vi "Get Raw Data.vi"(8 "error in (no error)":errorcluster, 11 "Red Pitaya Digitizer in":refnum<class "Red Pitaya Digitizer.lvclass">) -> (0 "error out":errorcluster, 1 "appended array":i16[][](array[numeric]), 3 "Red Pitaya Digitizer out":refnum<class "Red Pitaya Digitizer.lvclass">)   [LabVIEW 2021, in "Red Pitaya Digitizer.lvclass"]
uses:
  Red Pitaya Digitizer.lvclass
  C:/GitHub/NHMFL_Core/Libraries/Instruments/Pulse Driver/Lockin Digitizer Driver/Lockin Digitizer Driver.lvclass
  C:/GitHub/NHMFL_Core/Libraries/Instruments/Pulse Driver/Pulse Driver.lvclass
  Red Pitaya Digitizer.lvclass/Red Pitaya Digitizer.ctl
  Instruments/Pulse Driver/Pulse Driver.lvclass/Pulse Driver.ctl
  Read RP Instrument.vi
  Instruments/Pulse Driver/Read Pretrigger samples.vi
  Instruments/Pulse Driver/Read Samples per channel.vi
  Write RP Instrument.vi
  RP Core/RP Instrument/RP Instrument.lvclass
  Controls/Record Channels.ctl
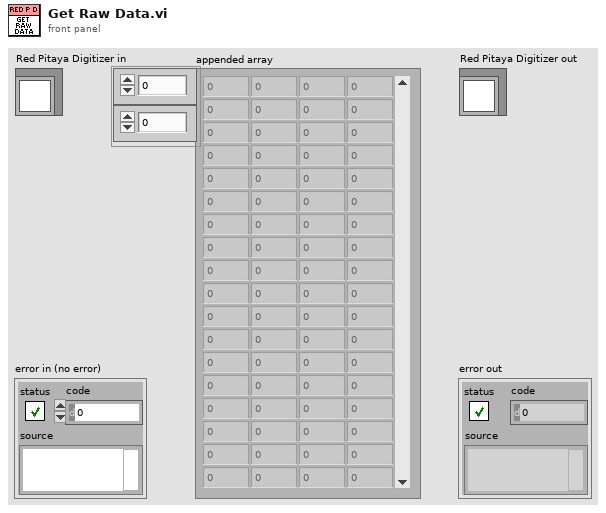
[diagram p1: front panel]
types:
  T1 = typedef "Record Channels.ctl" = enum16{"NONE", "FIRST", "SECOND", "BOTH"}
  T2 = enum16{"big-endian, network order", "native, host order", "little-endian"}
  T3 = typedef "Pusle Driver Configuration.ctl" = cluster{"Post-trigger delay":dbl, "Post-trigger duration":dbl, "Rate":dbl, "Ranges":dbl[], "Re-name channels":string[], "Active channels":string, "External clock":bool}
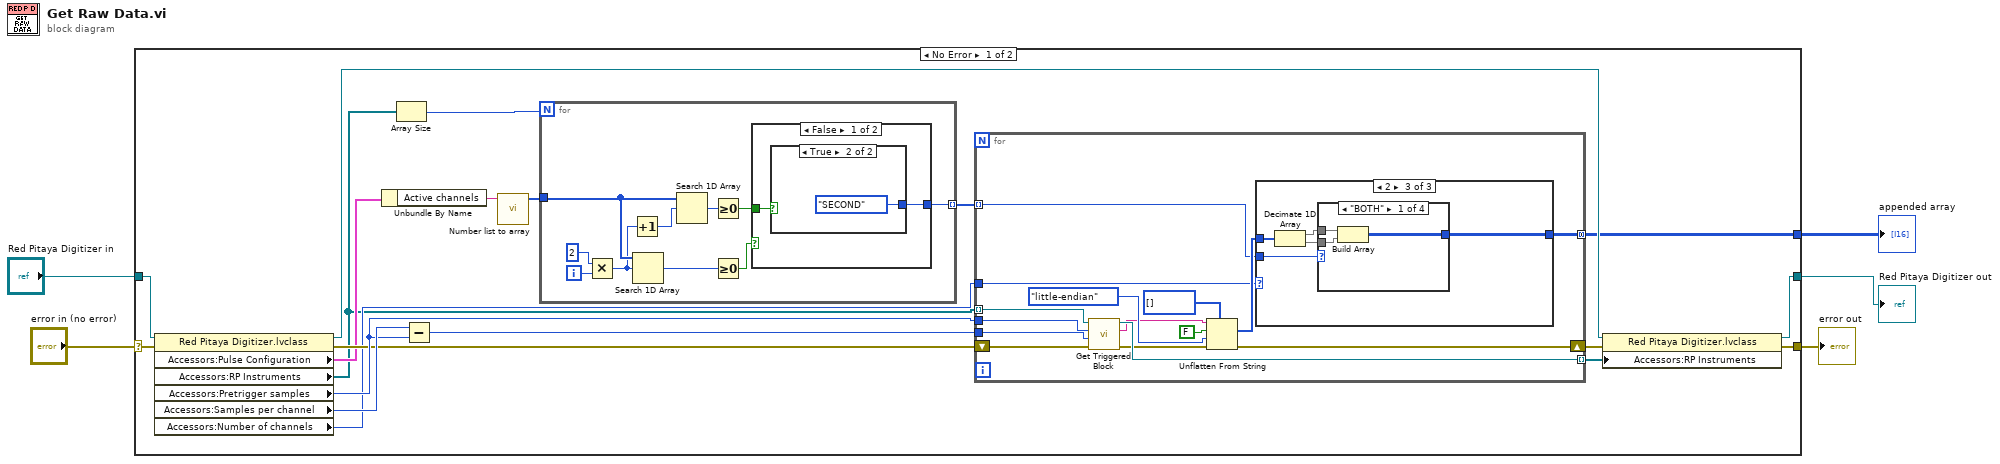
[diagram p0: block diagram]
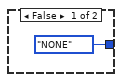
[diagram p2: hidden frame]
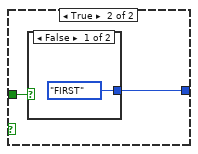
[diagram p3: hidden frame]
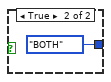
[diagram p4: hidden frame]
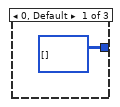
[diagram p5: hidden frame]
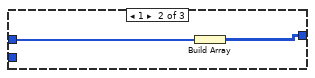
[diagram p6: hidden frame]
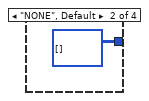
[diagram p7: hidden frame]
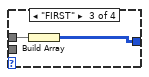
[diagram p8: hidden frame]
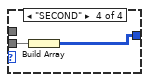
[diagram p9: hidden frame]
diagram:
  n1 = case shown="No Error" "error in (no error)" {
    selector: "error in (no error)" -> [w17 w75]
    tunnel: [w13 w75] -> w4
    tunnel: [w16 w74] -> w2
    tunnel: "Red Pitaya Digitizer in" -> [w18 w74]
    tunnel: [w15 _] -> w1
    frame No Error {
      n2 = property class="Red Pitaya Digitizer.lvclass"(reference=w18, error in=w17) -> (reference out=w24:refnum<class "Red Pitaya Digitizer.lvclass">, error out=w20:errorcluster, "Accessors:Pulse Configuration"=w11:T3, "Accessors:RP Instruments"=w9:refnum<class "RP Instrument.lvclass">[], "Accessors:Pretrigger samples"=w22:i32, "Accessors:Samples per channel"=w23:i32, "Accessors:Number of channels"=w12:i32)
      n3 = Unbundle By Name(w11) -> ("Active channels"=w10:string)
      n4 = Array Size(array=w9) -> (size(s)=w8:i32)
      n5 = Subtract(x=w23, y=w22) -> (x-y=w21:i32)
      n6 = call "Number list to array.vi"("Number list"=w10) -> ("Number list array"=w7:i32[])  [unwired: 8 in, 2 out]
      n7 = for {
        N: w8 -> [_]
        tunnel: w7 -> [w32]
        tunnel: [w27] -> w6 mode=indexing
        i -> [w34]
        n8 = Multiply(x=2, y=w34) -> (x*y=w26:i32)
        n9 = Increment(x=w26) -> (x+1=w25:i32)
        n10 = Search 1D Array(1D array=w32, element=w26) -> (index of element=w31:i32)  [unwired: 1 in]
        n11 = Search 1D Array(1D array=w32, element=w25) -> (index of element=w30:i32)  [unwired: 1 in]
        n12 = Greater Or Equal To 0?(x=w30) -> (x >= 0?=w28:bool)
        n13 = Greater Or Equal To 0?(x=w31) -> (x >= 0?=w29:bool)
        n14 = case shown="False" w29 {
          tunnel: w28 -> [w36 w40]
          tunnel: [w35 w39] -> w27
          frame False {
            n15 = case shown="True" w36 {
              tunnel: [Record_Channels."NONE" Record_Channels."SECOND"] -> w35
              frame False {
              }
              frame True {
              }
            }
          }
          frame True {
            n16 = case shown="False" w40 {
              tunnel: [Record_Channels."FIRST" Record_Channels."BOTH"] -> w39
              frame False {
              }
              frame True {
              }
            }
          }
        }
      }
      n17 = for {
        tunnel: w9 -> [w57] mode=indexing
        tunnel: w22 -> [w56]
        tunnel: w21 -> [w55]
        tunnel: [w53] -> w19 mode=indexing
        tunnel: [w47] -> w15 mode=concatenating
        shift-right: [w45] -> w14
        shift-left: w20 -> [w54]
        tunnel: w12 -> [w44]
        tunnel: w6 -> [w43] mode=indexing
        n18 = call-dynamic "Get Triggered Block.vi"("error in (no error)"=w54, "Post-trigger points"=w55, "Pre-trigger points"=w56, "RP Instrument in"=w57) -> ("error out"=w46:errorcluster, "Data out"=w48:string, "RP Instrument out"=w53:refnum<class "RP Instrument.lvclass">)  [unwired: 5 in]
        n19 = Unflatten From String(type=i16[] [], binary string=w48, data includes array or string size? (T)=FALSE, byte order (0:big-endian, network order)=T2."little-endian", error in (no error)=w46) -> (value=w49:i16[], error out=w45:errorcluster)  [unwired: 1 out]
        n20 = case shown="2" w44 {
          tunnel: w49 -> [_ w59 w64]
          tunnel: [i16[][] [] w60 w62] -> w47
          tunnel: w43 -> [_ _ w61]
          frame 0, Default {
          }
          frame 1 {
            n21 = Build Array(w59) -> (w60:i16[][])
          }
          frame 2 {
            n22 = Decimate 1D Array(w64) -> (w63:i16[], w65:i16[])
            n23 = case shown="\"BOTH\"" w61 {
              tunnel: w65 -> [w68 _ _ w72]
              tunnel: w63 -> [w67 _ w71 _]
              tunnel: [w66 i16[][] [] w70 w73] -> w62
              frame "BOTH" {
                n24 = Build Array(w67, w68) -> (w66:i16[][])
              }
              frame "NONE", Default {
              }
              frame "FIRST" {
                n25 = Build Array(w71) -> (w70:i16[][])
              }
              frame "SECOND" {
                n26 = Build Array(w72) -> (w73:i16[][])
              }
            }
          }
        }
      }
      n27 = property class="Red Pitaya Digitizer.lvclass"(reference=w24, error in=w14, "Accessors:RP Instruments"=w19) -> (reference out=w16:refnum<class "Red Pitaya Digitizer.lvclass">, error out=w13:errorcluster)
    }
    frame Error {
    }
  }
  "error out" <- w4
  "Red Pitaya Digitizer out" <- w2
  "appended array" <- w1
